vi "Exercise 3-1.vi"() -> ()   [LabVIEW 2014]
panel:
  out "Warning?":bool
  out "Warning Text":string
  in  "Min Temp":dbl
  in  "Max Temp":dbl
  in  "Current Temp":dbl
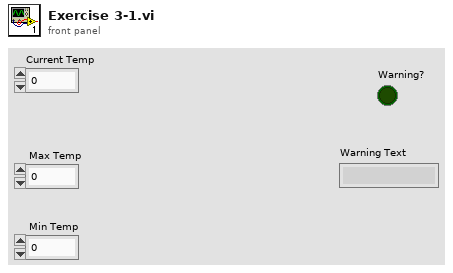
[diagram p1: front panel]
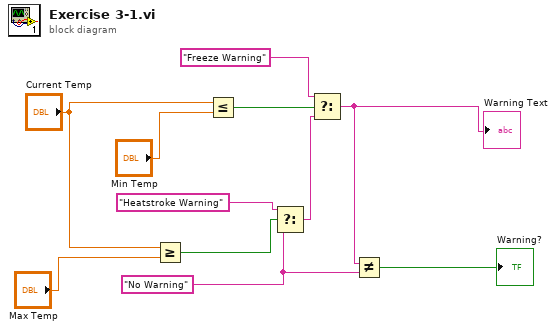
[diagram p0: block diagram]
diagram:
  w3 = "No Warning"
  n1 = Greater Or Equal?(x="Current Temp", y="Max Temp") -> (x >= y?=w8:bool)
  n2 = Less Or Equal?(x="Current Temp", y="Min Temp") -> (x <= y?=w6:bool)
  n3 = Select(t="Heatstroke Warning", s=w8, f=w3) -> (s? t:f=w5:string)
  n4 = Select(t="Freeze Warning", s=w6, f=w5) -> (s? t:f=w2:string)
  "Warning Text" <- w2
  n5 = Not Equal?(x=w2, y=w3) -> (x != y?=→"Warning?":bool)
